vi "Execute Query.vi"(8 "error in (no error)":errorcluster, 9 "connection reference in":T1, 10 "reference in":refnum<vi>, 11 "MulticolumnListbox in":refnum<vi>) -> (0 "error out":errorcluster, 3 "Refnum out":T1)   [LabVIEW 2018]
uses:
  <vilib>/addons/database/Connection.llb/Conn ObjectReference.ctl
  <vilib>/addons/database/Connection.llb/Conn Execute.vi
  <vilib>/addons/database/Recordset.llb/Rec Fetch Recordset Data (R).vi
  <vilib>/addons/database/_DB Variant To Data/Database Variant To Data.xnode
  <vilib>/addons/database/Recordset.llb/Rec Destroy - Connection.vi
  <vilib>/addons/database/NI_Database_API.lvlib
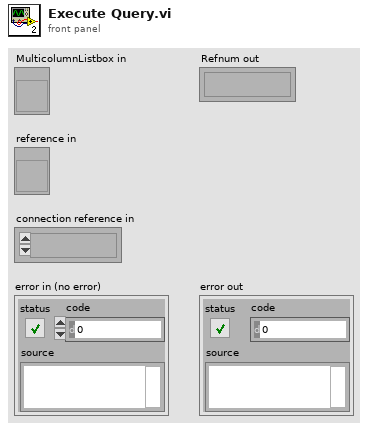
[diagram p1: front panel]
types:
  T1 = typedef "NI_Database_API.lvlib/Conn ObjectReference.ctl" = refnum<k1>
  T2 = typedef "NI_Database_API.lvlib/Rec ObjectReference.ctl" = refnum<k1>
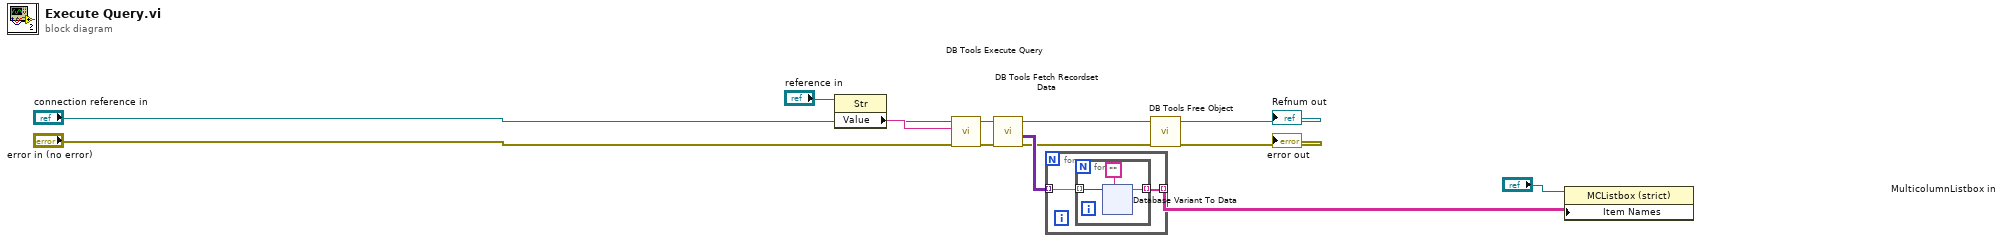
[diagram p0: block diagram]
diagram:
  n1 = property class="Str"(reference="reference in") -> ("Value"=w13:string)  [unwired: 1 in, 2 out]
  n2 = call-poly <vilib>:"DB Tools Execute Query.vi"("error in (no error)"="error in (no error)", "SQL query"=w13, "connection reference"="connection reference in") -> ("error out"=w7:errorcluster, "recordset reference"=w8:T2)  [unwired: 5 in]
  n3 = call-poly <vilib>:"DB Tools Fetch Recordset Data.vi"("error in (no error)"=w7, "recordset reference"=w8) -> ("error out"=w3:errorcluster, "recordset data"=w6:variant[][], "recordset reference out"=w4:T2)  [unwired: 3 in]
  n4 = for {
    tunnel: w6 -> [w15] mode=indexing
    tunnel: [w14] -> w5 mode=indexing
    n5 = for {
      tunnel: w15 -> [w18] mode=indexing
      tunnel: [w17] -> w14 mode=indexing
      n6 = xnode "Database Variant To Data"("database variant"=w18, "type"="") -> ("data"=w17:string)  [unwired: 1 in, 1 out]
    }
  }
  n7 = call-poly <vilib>:"DB Tools Free Object.vi"("error in (no error)"=w3, "recordset reference"=w4) -> ("error out"=→"error out":errorcluster, "connection reference"=→"Refnum out":T1)  [unwired: 8 in]
  n8 = property on="Property Node" class="MCListbox (strict)"(reference="MulticolumnListbox in", "Item Names"=w5) -> ()  [unwired: 1 in, 2 out]
